vi "ExposeMakeObjectMapNamepthData.vi"(0 "ObjectMapType":T3, 5 "namepath":string, 9 "value":variant, 11 "Labview Contriner type":T1) -> (4 "MatlabDataBundle":T2)   [LabVIEW 2017]
uses:
  ExposeMapperDataTypeEnum.ctl
  ExposeObjectMapNamepathData.ctl
  ExposeObjectMapContainerTypeEnum.ctl
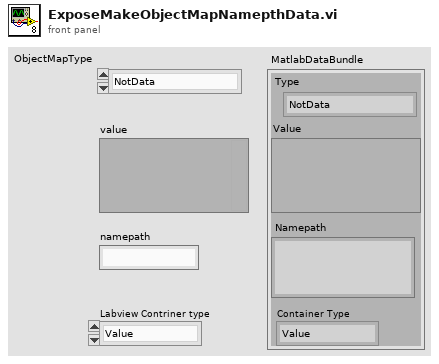
[diagram p1: front panel]
types:
  T1 = typedef "ExposeObjectMapContainerTypeEnum.ctl" = enum16{"Value", "Array", "Waveform", "NetContainer"}
  T2 = typedef "ExposeObjectMapNamepathData.ctl" = cluster{"Type":T3, "Value":variant, "Namepath":string, "Container Type":T1}
  T3 = typedef "ExposeMapperDataTypeEnum.ctl" = enum16{"NotData", "int8", "byte", "int16", "uint16", "int32", "uint32", "int64", "uint64", "Single", "Double", "String", "Boolean", "Container"}
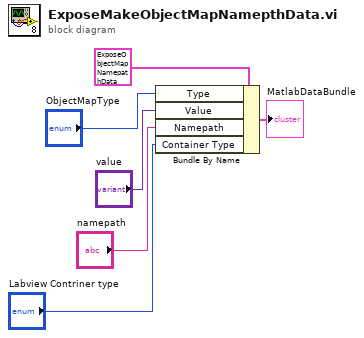
[diagram p0: block diagram]
diagram:
  n1 = Bundle By Name(cluster=T2 {"Type"=enum."NotData", "Value"=variant, "Namepath"="", "Container Type"=enum."Value"} ("input cluster"), "Type"="ObjectMapType", "Value"="value", "Namepath"="namepath", "Container Type"="Labview Contriner type") -> (→"MatlabDataBundle":T2)
